vi "Test RC.vi"(8 "error in (no error)":errorcluster, 11 "RC Type":T1=enum."ZMQ") -> (0 "error out":errorcluster)   [LabVIEW 2019]
uses:
  lvsrc/SMOs/RemoteControl/Typedefs/RC Com Type--enum.ctl
  <vilib>/addons/_JKI Toolkits/Caraya/classes/Assert/Assert Not Error.vi
  lvsrc/SMOs/RemoteControl/RemoteControl.lvclass
  <vilib>/addons/_JKI Toolkits/Caraya/classes/Assert/Assert.lvclass
  <vilib>/addons/_JKI Toolkits/Caraya/classes/Test/Test.lvclass
panel:
  # "1. Choose RC Type\n2. Run This VI\n3. An orange server will open. Three pink clients will then open. Watch the messasges.\n4. When you are satisfied:\n- first stop the clients and\n- then stop the server."
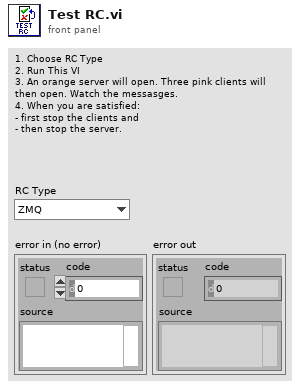
[diagram p1: front panel]
types:
  T1 = typedef "RemoteControl.lvclass/RC Com Type--enum.ctl" = enum16{"RC", "STM", "ZMQ"}
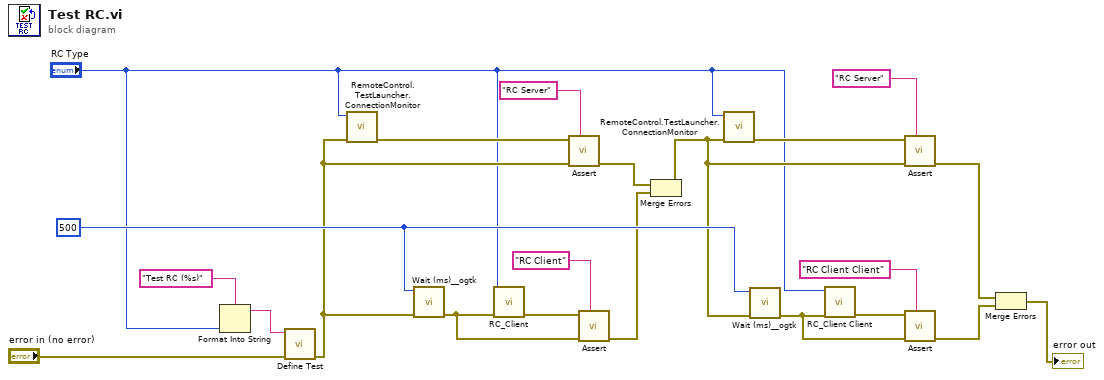
[diagram p0: block diagram]
diagram:
  w11 = u32 500 ("milliseconds to wait")
  n1 = Format Into String(format string="Test RC (%s)", "RC Type") -> (resulting string=w20:string)  [unwired: 2 in, 1 out]
  n2 = call <vilib>:"Define Test.vi"("error in (no error)"="error in (no error)", "Label (VI Title)"=w20) -> ("error out"=w3:errorcluster)  [unwired: 9 in]
  n3 = call "RemoteControl.TestLauncher.ConnectionMonitor.vi"("error in (no error)"=w3, "RC COM Type"="RC Type") -> ("error out"=w18:errorcluster)  [unwired: 9 in]
  n4 = call <userlib>:"Wait (ms)__ogtk.vi"("error in (no error)"=w3, "milliseconds to wait"=w11) -> ("error out"=w16:errorcluster)  [unwired: 8 in, 1 out]
  n5 = call "RC_Client.vi"("error in (no error)"=w16, "RC Type"="RC Type") -> ("error out"=w17:errorcluster)  [unwired: 9 in]
  n6 = call-poly <vilib>:"Assert.vi"("Label"="RC Server", "error in (no error)"=w3, "Not Error?"=w18) -> ("error out"=w10:errorcluster)  [unwired: 8 in]
  n7 = call-poly <vilib>:"Assert.vi"("Label"="RC Client", "error in (no error)"=w16, "Not Error?"=w17) -> ("error out"=w9:errorcluster)  [unwired: 8 in]
  n8 = Merge Errors(w10, w9) -> (w4:errorcluster)
  n9 = call "RemoteControl.TestLauncher.ConnectionMonitor.vi"("error in (no error)"=w4, "RC COM Type"="RC Type") -> ("error out"=w13:errorcluster)  [unwired: 9 in]
  n10 = call <userlib>:"Wait (ms)__ogtk.vi"("error in (no error)"=w4, "milliseconds to wait"=w11) -> ("error out"=w15:errorcluster)  [unwired: 8 in, 1 out]
  n11 = call "RC_Client Client.vi"("error in (no error)"=w15, "RC Type"="RC Type") -> ("error out"=w14:errorcluster)  [unwired: 9 in]
  n12 = call-poly <vilib>:"Assert.vi"("Label"="RC Server", "error in (no error)"=w4, "Not Error?"=w13) -> ("error out"=w2:errorcluster)  [unwired: 8 in]
  n13 = call-poly <vilib>:"Assert.vi"("Label"="RC Client Client", "error in (no error)"=w15, "Not Error?"=w14) -> ("error out"=w12:errorcluster)  [unwired: 8 in]
  n14 = Merge Errors(w2, w12) -> (→"error out":errorcluster)
